vi "Read Thermo Setting.vi"(8 "error in (no error)":errorcluster, 11 "Thermo Instrument configuration":refnum<class "Thermo configuration.lvclass">) -> (0 "error out":errorcluster, 2 "Thermo Setting":T1={"Numeric"=0.5, "Combo"="", "String"="", "Boolean"=FALSE} {"Numeric" format="%#_f"}, 3 "Thermo Instrument configuration out":refnum<class "Thermo configuration.lvclass">)   [LabVIEW 2025, in "Thermo.lvlib" / "Thermo configuration.lvclass"]
uses:
  Thermo configuration.lvclass
  Thermo configuration.lvclass/Thermo configuration.ctl
  Thermo Setting.ctl
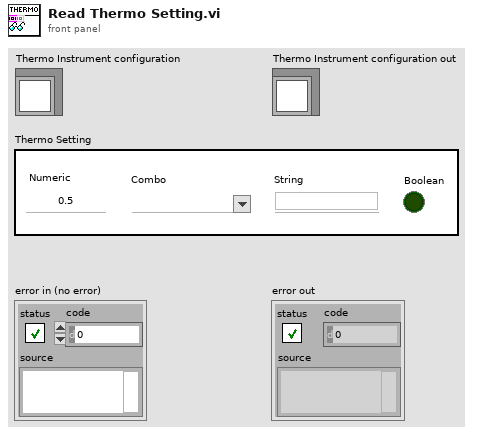
[diagram p1: front panel]
types:
  T1 = typedef "Thermo.lvlib/Thermo configuration.lvclass/Thermo Setting.ctl" = cluster{"Numeric":dbl, "Combo":string, "String":string, "Boolean":bool}
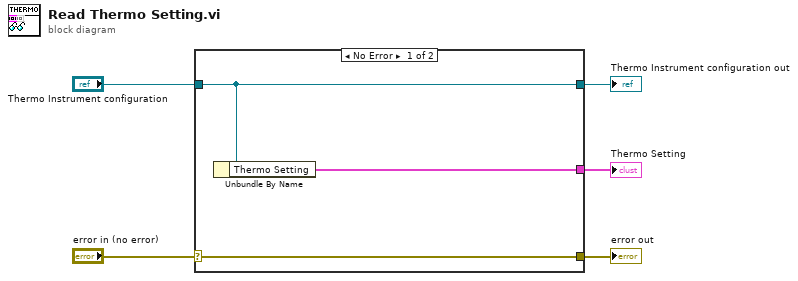
[diagram p0: block diagram]
diagram:
  n1 = case shown="No Error" "error in (no error)" {
    selector: "error in (no error)" -> [w8 w9]
    tunnel: [w8 w9] -> w4
    tunnel: [w7 w10] -> w2
    tunnel: "Thermo Instrument configuration" -> [w7 w10]
    tunnel: [w6 _] -> w1
    frame No Error {
      n2 = Unbundle By Name(w7) -> ("Thermo Setting"=w6:T1)
    }
    frame Error {
    }
  }
  "error out" <- w4
  "Thermo Instrument configuration out" <- w2
  "Thermo Setting" <- w1
